vi "Intensity Graph to XY Graph (Horizontal) (by ref).vi"(8 "error in (no error)":errorcluster, 11 "graph_utilities in":refnum<class "graph_utilities.lvclass">) -> (0 "error out":errorcluster, 3 "graph_utilities out":refnum<class "graph_utilities.lvclass">)   [LabVIEW 2019, in "graph_utilities.lvclass"]
doc: "Converts an Intensity Graph into a sequence of plots on a XY Graph.\n\nThe x-axis of the XY Graph will be equal to the x-axis of the Intensity Graph."
uses:
  graph_utilities.lvclass
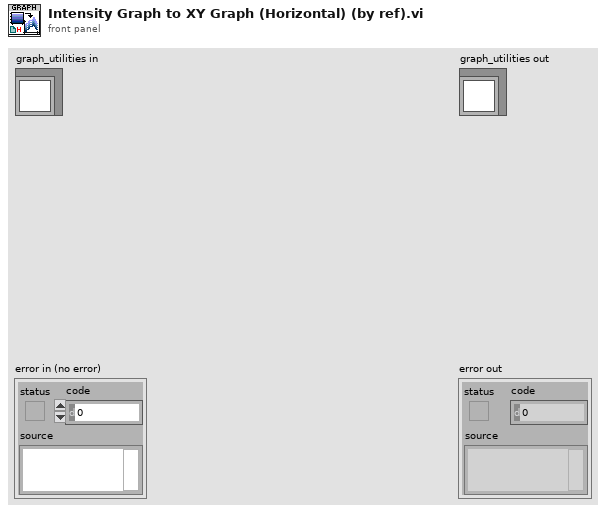
[diagram p1: front panel]
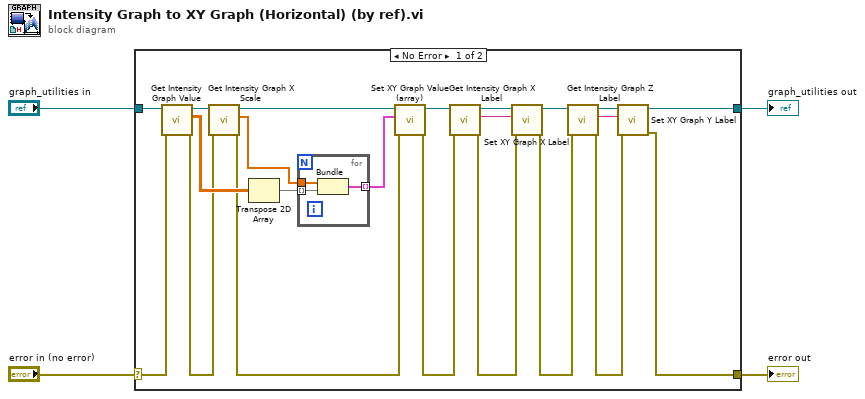
[diagram p0: block diagram]
diagram:
  n1 = case shown="No Error" "error in (no error)" {
    selector: "error in (no error)" -> [w11 w31]
    tunnel: [w8 w31] -> w3
    tunnel: [w9 w30] -> w1
    tunnel: "graph_utilities in" -> [w26 w30]
    frame No Error {
      n2 = call "Get Intensity Graph Value.vi"("error in (no error)"=w11, "graph_utilities in"=w26) -> ("error out"=w10:errorcluster, "Value"=w25:dbl[][], "graph_utilities out"=w12:refnum<class "graph_utilities.lvclass">)  [unwired: 7 in]
      n3 = call "Get Intensity Graph X Scale.vi"("error in (no error)"=w10, "graph_utilities in"=w12) -> ("error out"=w23:errorcluster, "X Scale"=w5:dbl[], "graph_utilities out"=w24:refnum<class "graph_utilities.lvclass">)  [unwired: 6 in, 1 out]
      n4 = Transpose 2D Array(2D array=w25) -> (transposed array=w7:dbl[][])
      n5 = for {
        tunnel: w7 -> [w28] mode=indexing
        tunnel: w5 -> [w29]
        tunnel: [w27] -> w6 mode=indexing
        n6 = Bundle("X Scale"=w29, w28) -> (w27:cluster{"X Scale":dbl[], dbl[]})  [unwired: 1 in]
      }
      n7 = call "Set XY Graph Value (array).vi"("error in (no error)"=w23, "XY-data"=w6, "graph_utilities in"=w24) -> ("error out"=w15:errorcluster, "graph_utilities out"=w16:refnum<class "graph_utilities.lvclass">)  [unwired: 7 in]
      n8 = call "Get Intensity Graph X Label.vi"("error in (no error)"=w15, "graph_utilities in"=w16) -> ("error out"=w14:errorcluster, "X Label"=w22:string, "graph_utilities out"=w17:refnum<class "graph_utilities.lvclass">)  [unwired: 7 in]
      n9 = call "Set XY Graph X Label.vi"("error in (no error)"=w14, "X Label"=w22, "graph_utilities in"=w17) -> ("error out"=w18:errorcluster, "graph_utilities out"=w19:refnum<class "graph_utilities.lvclass">)  [unwired: 7 in]
      n10 = call "Get Intensity Graph Z Label.vi"("error in (no error)"=w18, "graph_utilities in"=w19) -> ("error out"=w13:errorcluster, "Z Label"=w21:string, "graph_utilities out"=w20:refnum<class "graph_utilities.lvclass">)  [unwired: 7 in]
      n11 = call "Set XY Graph Y Label.vi"("error in (no error)"=w13, "Y Label"=w21, "graph_utilities in"=w20) -> ("error out"=w8:errorcluster, "graph_utilities out"=w9:refnum<class "graph_utilities.lvclass">)  [unwired: 7 in]
    }
    frame Error {
    }
  }
  "error out" <- w3
  "graph_utilities out" <- w1
